vi "UI - Header.vi"(5 "Term (Methods)":string="Methods", 7 "Msg Chain":string, 8 "error in (no error)":errorcluster {"code" format="Error %.0f"}, 11 "VIDoc Printer - Confluence In":refnum<class "VIDoc Printer - Confluence.lvclass">) -> (0 "error out":errorcluster {"code" format="Error %.0f"}, 3 "VIDoc Printer - Confluence Out":refnum<class "VIDoc Printer - Confluence.lvclass">)   [LabVIEW 2023, in "VIDoc Printer - Confluence.lvlib" / "VIDoc Printer - Confluence.lvclass"]
uses:
  VIDoc Printer - Confluence.lvclass
  VIDoc Printer - Confluence.lvclass/VIDoc Printer - Confluence.ctl
  Confluence Formatting/Confluence Formatting.lvlib
  Confluence Formatting/Types/Format Combo Box.ctl
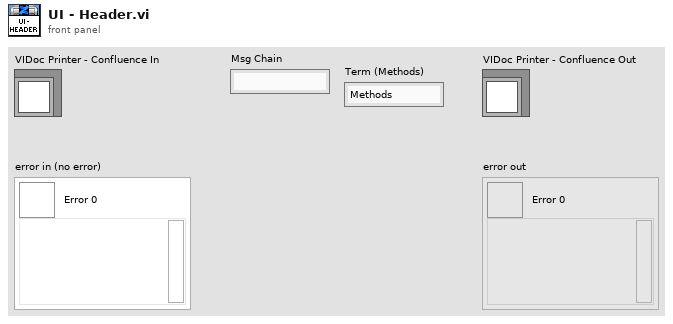
[diagram p1: front panel]
types:
  T1 = typedef "Confluence Formatting.lvlib/Format Combo Box.ctl" = string
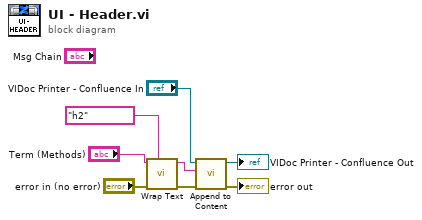
[diagram p0: block diagram]
diagram:
  n1 = call "Wrap Text.vi"("Formatting"=T1 "h2", "Error in"="error in (no error)", "String"="Term (Methods)") -> ("Error out"=w6:errorcluster, "Wrapped String"=w2:string)  [unwired: 7 in]
  n2 = call "Append to Content.vi"("error in (no error)"=w6, "Content"=w2, "VIDoc Printer - Confluence In"="VIDoc Printer - Confluence In") -> ("error out"=→"error out":errorcluster, "VIDoc Printer - Confluence Out"=→"VIDoc Printer - Confluence Out":refnum<class "VIDoc Printer - Confluence.lvclass">)  [unwired: 7 in]
